vi "WILT Agilent Valve Control.vi"(0 "Station In":string="33", 1 "Agilent Channels In":T4[](array[typedef])=[{"Channel"="301", "Station"="1", "Label"="Water Valve", "Agilent Station"="2", "Data"=0.0}, {"Channel"="302", "Station"="2", "Label"="Water Valve", "Agilent Station"="2", "Data"=0.0}, {"Channel"="303", "Station"="3", "Label"="Water Valve", "Agilent Station"="2", "Data"=0.0}, {"Channel"="304", "Station"="4", "Label"="Water Valve", "Agilent Station"="2", "Data"=0.0}, {"Channel"="305", "Station"="5", "Label"="Water Valve", "Agilent Station"="2", "Data"=0.0}, {"Channel"="306", "Station"="6", "Label"="Water Valve", "Agilent Station"="2", "Data"=0.0}, {"Channel"="307", "Station"="7", "Label"="Water Valve", "Agilent Station"="2", "Data"=0.0}, {"Channel"="308", "Station"="8", "Label"="Water Valve", "Agilent Station"="2", "Data"=0.0}, {"Channel"="309", "Station"="9", "Label"="Water Valve", "Agilent Station"="2", "Data"=0.0}, {"Channel"="310", "Station"="10", "Label"="Water Valve", "Agilent Station"="2", "Data"=0.0}, {"Channel"="311", "Station"="11", "Label"="Water Valve", "Agilent Station"="2", "Data"=0.0}, {"Channel"="312", "Station"="12", "Label"="Water Valve", "Agilent Station"="2", "Data"=0.0}, {"Channel"="313", "Station"="13", "Label"="Water Valve", "Agilent Station"="2", "Data"=0.0}, {"Channel"="314", "Station"="14", "Label"="Water Valve", "Agilent Station"="2", "Data"=0.0}, {"Channel"="315", "Station"="15", "Label"="Water Valve", "Agilent Station"="2", "Data"=0.0}, {"Channel"="316", "Station"="16", "Label"="Water Valve", "Agilent Station"="2", "Data"=0.0}, {"Channel"="317", "Station"="17", "Label"="Water Valve", "Agilent Station"="2", "Data"=0.0}, {"Channel"="318", "Station"="18", "Label"="Water Valve", "Agilent Station"="2", "Data"=0.0}, {"Channel"="319", "Station"="19", "Label"="Water Valve", "Agilent Station"="2", "Data"=0.0}, {"Channel"="320", "Station"="20", "Label"="Water Valve", "Agilent Station"="2", "Data"=0.0}, {"Channel"="101", "Station"="21", "Label"="Water Valve", "Agilent Station"="3", "Data"=0.0}, {"Channel"="102", "Station"="22", "Label"="Water Valve", "Agilent Station"="3", "Data"=0.0}, {"Channel"="103", "Station"="23", "Label"="Water Valve", "Agilent Station"="3", "Data"=0.0}, {"Channel"="104", "Station"="24", "Label"="Water Valve", "Agilent Station"="3", "Data"=0.0}, {"Channel"="105", "Station"="25", "Label"="Water Valve", "Agilent Station"="3", "Data"=0.0}, {"Channel"="106", "Station"="26", "Label"="Water Valve", "Agilent Station"="3", "Data"=0.0}, {"Channel"="107", "Station"="27", "Label"="Water Valve", "Agilent Station"="3", "Data"=0.0}, {"Channel"="108", "Station"="28", "Label"="Water Valve", "Agilent Station"="3", "Data"=0.0}, {"Channel"="109", "Station"="29", "Label"="Water Valve", "Agilent Station"="3", "Data"=0.0}, {"Channel"="110", "Station"="30", "Label"="Water Valve", "Agilent Station"="3", "Data"=0.0}, {"Channel"="111", "Station"="31", "Label"="Water Valve", "Agilent Station"="3", "Data"=0.0}, {"Channel"="112", "Station"="32", "Label"="Water Valve", "Agilent Station"="3", "Data"=0.0}, {"Channel"="101", "Station"="33", "Label"="Water Valve", "Agilent Station"="5", "Data"=0.0}, {"Channel"="102", "Station"="34", "Label"="Water Valve", "Agilent Station"="5", "Data"=0.0}, {"Channel"="103", "Station"="35", "Label"="Water Valve", "Agilent Station"="5", "Data"=0.0}, {"Channel"="104", "Station"="36", "Label"="Water Valve", "Agilent Station"="5", "Data"=0.0}, {"Channel"="105", "Station"="37", "Label"="Water Valve", "Agilent Station"="5", "Data"=0.0}, {"Channel"="106", "Station"="38", "Label"="Water Valve", "Agilent Station"="5", "Data"=0.0}, {"Channel"="107", "Station"="39", "Label"="Water Valve", "Agilent Station"="5", "Data"=0.0}, {"Channel"="108", "Station"="40", "Label"="Water Valve", "Agilent Station"="5", "Data"=0.0}, {"Channel"="109", "Station"="41", "Label"="Water Valve", "Agilent Station"="5", "Data"=0.0}, {"Channel"="110", "Station"="42", "Label"="Water Valve", "Agilent Station"="5", "Data"=0.0}, {"Channel"="111", "Station"="43", "Label"="Water Valve", "Agilent Station"="5", "Data"=0.0}, {"Channel"="112", "Station"="44", "Label"="Water Valve", "Agilent Station"="5", "Data"=0.0}, {"Channel"="113", "Station"="45", "Label"="Water Valve", "Agilent Station"="5", "Data"=0.0}, {"Channel"="114", "Station"="46", "Label"="Water Valve", "Agilent Station"="5", "Data"=0.0}, {"Channel"="115", "Station"="47", "Label"="Water Valve", "Agilent Station"="5", "Data"=0.0}, {"Channel"="116", "Station"="48", "Label"="Water Valve", "Agilent Station"="5", "Data"=0.0}, {"Channel"="117", "Station"="49", "Label"="Water Valve", "Agilent Station"="5", "Data"=0.0}, {"Channel"="118", "Station"="50", "Label"="Water Valve", "Agilent Station"="5", "Data"=0.0}, {"Channel"="119", "Station"="51", "Label"="Water Valve", "Agilent Station"="5", "Data"=0.0}, {"Channel"="120", "Station"="52", "Label"="Water Valve", "Agilent Station"="5", "Data"=0.0}, {"Channel"="201", "Station"="53", "Label"="Water Valve", "Agilent Station"="5", "Data"=0.0}, {"Channel"="202", "Station"="54", "Label"="Water Valve", "Agilent Station"="5", "Data"=0.0}, {"Channel"="203", "Station"="55", "Label"="Water Valve", "Agilent Station"="5", "Data"=0.0}, {"Channel"="204", "Station"="56", "Label"="Water Valve", "Agilent Station"="5", "Data"=0.0}, {"Channel"="301", "Station"="21", "Label"="Start Button", "Agilent Station"="5", "Data"=0.0}, {"Channel"="302", "Station"="22", "Label"="Start Button", "Agilent Station"="5", "Data"=0.0}, {"Channel"="303", "Station"="23", "Label"="Start Button", "Agilent Station"="5", "Data"=0.0}, {"Channel"="304", "Station"="24", "Label"="Start Button", "Agilent Station"="5", "Data"=0.0}, {"Channel"="305", "Station"="25", "Label"="Start Button", "Agilent Station"="5", "Data"=0.0}, {"Channel"="306", "Station"="26", "Label"="Start Button", "Agilent Station"="5", "Data"=0.0}, {"Channel"="307", "Station"="27", "Label"="Start Button", "Agilent Station"="5", "Data"=0.0}, {"Channel"="308", "Station"="28", "Label"="Start Button", "Agilent Station"="5", "Data"=0.0}, {"Channel"="309", "Station"="29", "Label"="Start Button", "Agilent Station"="5", "Data"=0.0}, {"Channel"="310", "Station"="30", "Label"="Start Button", "Agilent Station"="5", "Data"=0.0}, {"Channel"="311", "Station"="31", "Label"="Start Button", "Agilent Station"="5", "Data"=0.0}, {"Channel"="312", "Station"="32", "Label"="Start Button", "Agilent Station"="5", "Data"=0.0}, {"Channel"="101", "Station"="33", "Label"="Start Button", "Agilent Station"="7", "Data"=0.0}, {"Channel"="102", "Station"="34", "Label"="Start Button", "Agilent Station"="7", "Data"=0.0}, {"Channel"="103", "Station"="35", "Label"="Start Button", "Agilent Station"="7", "Data"=0.0}, {"Channel"="104", "Station"="36", "Label"="Start Button", "Agilent Station"="7", "Data"=0.0}, {"Channel"="105", "Station"="37", "Label"="Start Button", "Agilent Station"="7", "Data"=0.0}, {"Channel"="106", "Station"="38", "Label"="Start Button", "Agilent Station"="7", "Data"=0.0}, {"Channel"="107", "Station"="39", "Label"="Start Button", "Agilent Station"="7", "Data"=0.0}, {"Channel"="108", "Station"="40", "Label"="Start Button", "Agilent Station"="7", "Data"=0.0}, {"Channel"="109", "Station"="41", "Label"="Start Button", "Agilent Station"="7", "Data"=0.0}, {"Channel"="110", "Station"="42", "Label"="Start Button", "Agilent Station"="7", "Data"=0.0}, {"Channel"="111", "Station"="43", "Label"="Start Button", "Agilent Station"="7", "Data"=0.0}, {"Channel"="112", "Station"="44", "Label"="Start Button", "Agilent Station"="7", "Data"=0.0}], 2 "Semaphore":T3[](array[typedef]), 3 "Search":T2="Water Valve", 5 "Open/Close (F:Close)":bool=TRUE, 11 "error in (no error)":errorcluster, 12 "Test Type":T1=enum."Full Valve Control", 13 "Number Of Cycles":i32, 14 "Cycle Time (mS)":u32=1000) -> (4 "Channel State?":string="1\n", 6 "Success":bool, 15 "error out":errorcluster)   [LabVIEW 2016]
uses:
  Type Definitions/WILT Agilent Channel Definition.ctl
  Type Definitions/WILT Switch Search.ctl
  Type Definitions/WILT Water Valve Test Type.ctl
  Drivers/Agilent 34972/Agilent 34970.lvlib
panel:
  out "Found Water Valve":bool
  out "Channel":string
  out "Agilent Station":string
  in  "Debug Reset":bool
  out "VISA resource name":refnum<visa-resource-name>="AGILENT5"
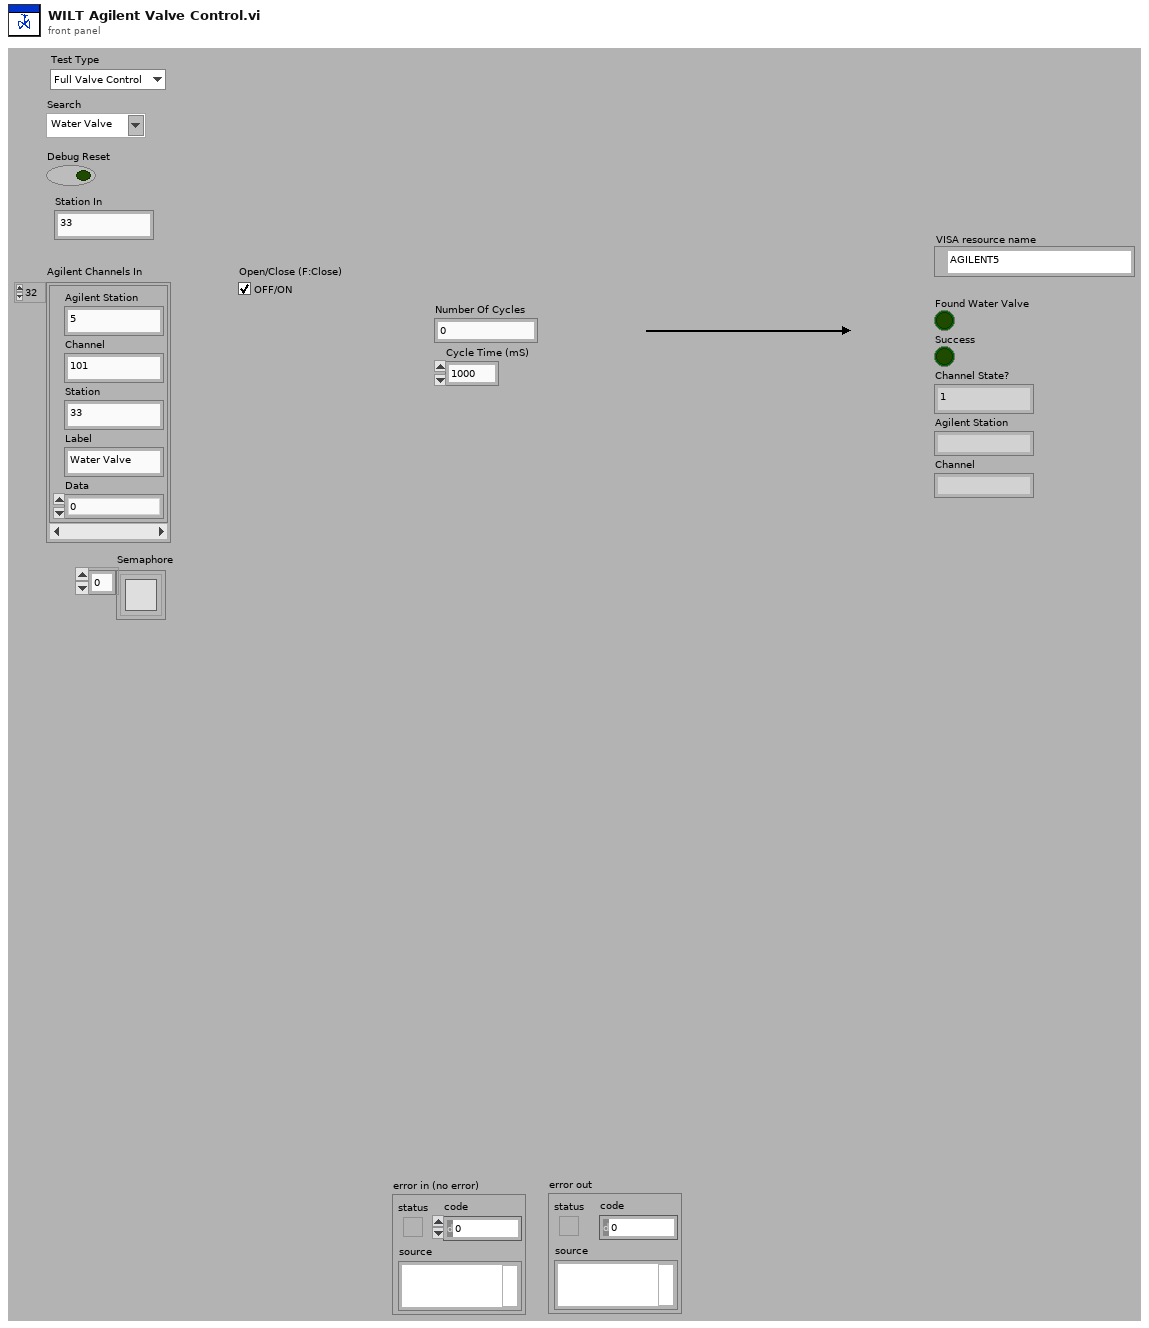
[diagram p1: front panel]
types:
  T1 = typedef "WILT Water Valve Test Type.ctl" = enum16{"Cycle Valve Control", "Full Valve Control"}
  T2 = typedef "WILT Switch Search.ctl" = string
  T3 = typedef "Semaphore RefNum" = refnum<k1>
  T4 = typedef "WILT Agilent Channel Definition.ctl" = cluster{"Channel":string, "Station":string, "Label":string, "Agilent Station":string, "Data":dbl}
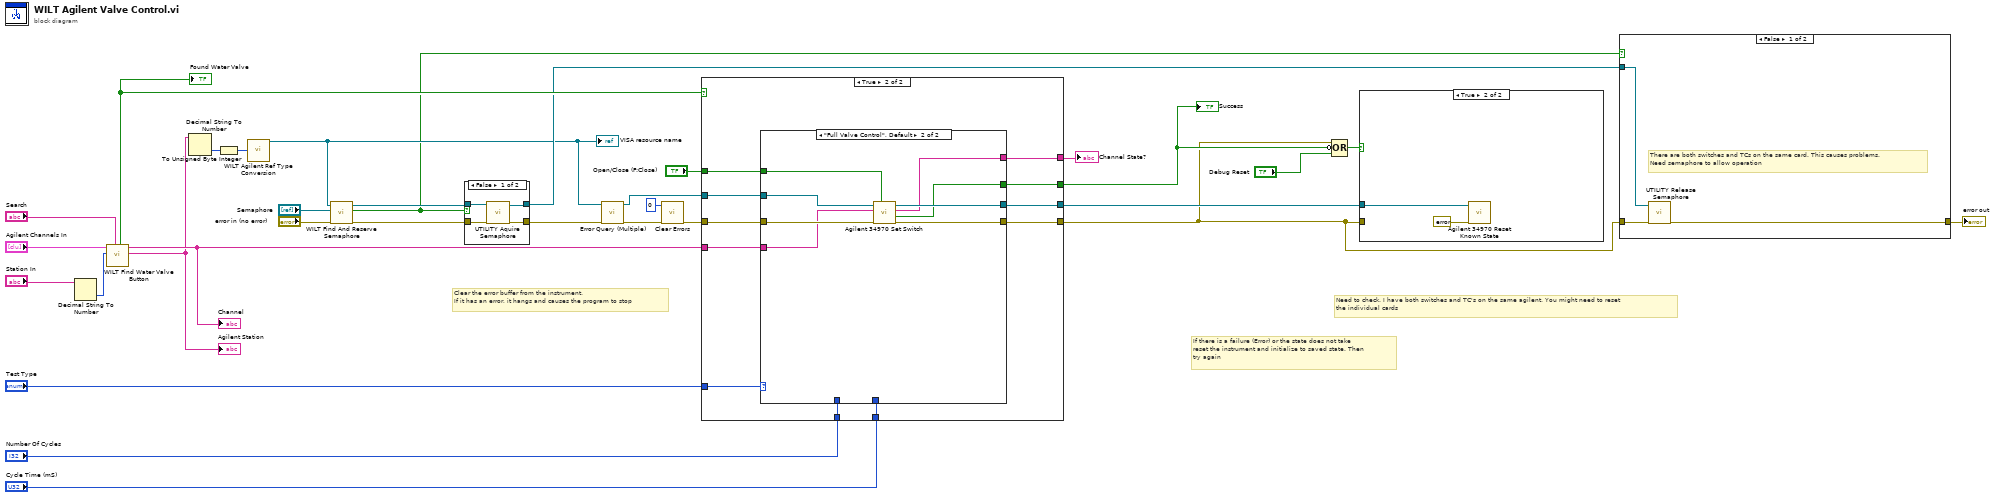
[diagram p0: block diagram]
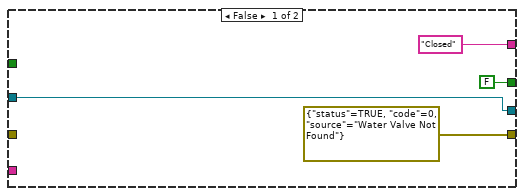
[diagram p5: hidden frame]
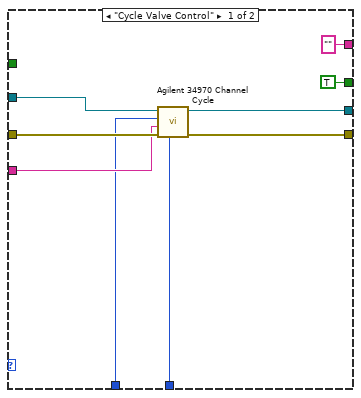
[diagram p6: hidden frame]
diagram:
  # "If there is a failure (Error) or the state does not take\nreset the instrument and initialize to saved state. Then\ntry again"
  # "Need to check. I have both switches and TC's on the same agilent. You might need to reset\nthe individual cards"
  # "Clear the error buffer from the instrument. \nIf it has an error, it hangs and causes the program to stop"
  n1 = Decimal String To Number(string="Station In") -> (number=w26:i32)  [unwired: 2 in, 1 out]
  n2 = call "WILT Find Water Valve Button.vi"("Search"="Search", "Station Number"=w26, "Agilent Valve and Switch Locations"="Agilent Channels In") -> ("Agilent Station"=w23:string, "Channel"=w24:string, "Found Water Valve"=w25:bool)  [unwired: 4 in, 2 out]
  "Agilent Station" <- w23
  "Channel" <- w24
  "Found Water Valve" <- w25
  n3 = Decimal String To Number(string=w23) -> (number=w32:i32)  [unwired: 2 in, 1 out]
  n4 = To Unsigned Byte Integer(number=w32) -> (unsigned 8bit integer=w31:u8)
  n5 = call "WILT Agilent Ref Type Conversion.vi"("Agilent Ref"=w31) -> ("VISA resource name"=w11:refnum<visa-resource-name>)  [unwired: 14 in]
  "VISA resource name" <- w11
  n6 = call "WILT Find And Reserve Semaphore.vi"("error in (no error)"="error in (no error)", "Semaphore"="Semaphore", "VISA Refnum in"=w11) -> ("error out"=w8:errorcluster, "Skip Semaphore"=w7:bool, "Refnum out"=w10:T3)  [unwired: 6 in]
  n7 = case shown="False" w7 {
    tunnel: [w36 w38] -> w15
    tunnel: [w35 w37] -> w13
    tunnel: w10 -> [w34 w37]
    tunnel: w8 -> [w33 w38]
    frame False {
      n8 = call "UTILITY Aquire Semaphore.vi"("error in (no error)"=w33, "Refnum in"=w34) -> ("error out"=w36:errorcluster, "Refnum out"=w35:T3)  [unwired: 7 in, 1 out]
    }
    frame True {
    }
  }
  n9 = call "Error Query (Multiple).vi"("VISA Resource Name"=w11, "error in (no error)"=w15) -> ("VISA Resource Name Out"=w22:refnum<visa-resource-name>, "error out"=w21:errorcluster)  [unwired: 10 in, 2 out]
  n10 = call <vilib>:"Clear Errors.vi"("error in (no error)"=w21, "specific error code to clear (0: all)"=0) -> ("error out"=w20:errorcluster)  [unwired: 4 in, 1 out]
  n11 = case shown="True" w25 {
    tunnel: w22 -> [w39 w51]
    tunnel: "Open/Close (F:Close)" -> [_ w49]
    tunnel: w20 -> [_ w53]
    tunnel: [errorcluster {"status"=TRUE, "code"=0, "source"="Water Valve Not Found"} ("error out") w52] -> w6
    tunnel: w24 -> [_ w50]
    tunnel: [FALSE w46] -> w16
    tunnel: ["Closed" w47] -> w29
    tunnel: [w39 w48] -> w18
    tunnel: "Number Of Cycles" -> [_ w45]
    tunnel: "Cycle Time (mS)" -> [_ w44]
    tunnel: "Test Type" -> [_ w43]
    frame False {
    }
    frame True {
      n12 = case shown="\"Full Valve Control\", Default" w43 {
        tunnel: w53 -> [w62 w70]
        tunnel: [w61 w69] -> w52
        tunnel: w51 -> [w60 w68]
        tunnel: w50 -> [w58 w67]
        tunnel: w49 -> [_ w66]
        tunnel: [w59 w65] -> w48
        tunnel: ["" ("Channel State?") w64] -> w47
        tunnel: [TRUE ("Success") w63] -> w46
        tunnel: w45 -> [w57 _]
        tunnel: w44 -> [w56 _]
        frame "Cycle Valve Control" {
          n13 = call "Agilent 34970 Channel Cycle.vi"("Cycle Time (mS)"=w56, "error in (no error)"=w62, "Channel"=w58, "Number Of Cycles"=w57, "VISA Refnum in"=w60) -> ("error out"=w61:errorcluster, "VISA Resource Name Out"=w59:refnum<visa-resource-name>)  [unwired: 5 in]
        }
        frame "Full Valve Control", Default {
          n14 = call "Agilent 34970 Set Switch.vi"("Open/Close (F:Close)"=w66, "error in (no error)"=w70, "Channel"=w67, "VISA Refnum in"=w68) -> ("error out"=w69:errorcluster, "Success"=w63:bool, "Channel State?"=w64:string, "VISA Resource Name Out"=w65:refnum<visa-resource-name>)  [unwired: 4 in]
        }
      }
    }
  }
  "Success" <- w16
  "Channel State?" <- w29
  n15 = Compound Arithmetic op=OR(w6, invert w16, "Debug Reset") -> (w19:bool)
  n16 = case shown="True" w19 {
    tunnel: w6 -> [_ _]
    tunnel: w18 -> [_ w72]
    frame False {
    }
    frame True {
      n17 = call "Agilent 34970 Reset Known State.vi"("Error In"=errorcluster {"status"=TRUE, "code"=0, "source"=""}, "VISA Refnum in"=w72) -> ()  [unwired: 9 in, 1 out]
    }
  }
  n18 = case shown="False" w7 {
    tunnel: w6 -> [w75 w76]
    tunnel: [w74 w76] -> w14
    tunnel: w13 -> [w73 _]
    frame False {
      # "There are both switches and TCs on the same card. This causes problems.\nNeed semaphore to allow operation"
      n19 = call "UTILITY Release Semaphore.vi"("error in (no error)"=w75, "Refnum in"=w73) -> ("error out"=w74:errorcluster)  [unwired: 9 in]
    }
    frame True {
    }
  }
  "error out" <- w14
